vi "Set Error Check.vi"(10 "Error Check":bool=TRUE, 11 "System no.":i32=1 min=1 step=1) -> ()   [LabVIEW 2026]
doc: "This VI enables the error check in Global1.vi for the selected System no."
uses:
  Global1.vi
panel:
  # "This vi enables the error check in Global1.vi for the selected system no."
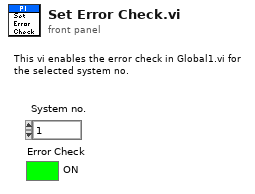
[diagram p1: front panel]
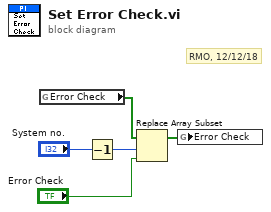
[diagram p0: block diagram]
diagram:
  # "RMO, 12/12/18"
  n1 = global read "Global1.vi" "Error Check"() -> (w5:bool[])
  n2 = Decrement(x="System no.") -> (x-1=w3:i32)
  n3 = Replace Array Subset(array=w5, new element="Error Check", index=w3) -> (w1:bool[])
  n4 = global write "Global1.vi" "Error Check"(w1) -> ()
